vi "Implementation of Fast imaq image encode and decode.vi"() -> ()   [LabVIEW 2020]
uses:
  <vilib>/vision/Image Controls.llb/IMAQ Image.ctl
  <vilib>/NI/Tools/String/Tools_String.lvlib
  <vilib>/Analysis/NI_AALBase.lvlib
panel:
  out "Percent":dbl
  out "length1":i32
  out "length2":i32
  in  "TIFF Options":T1={"Rows Per Strip"=0, "Photometric"=1, "Compression Type"=0} {"Compression Type" items=["None", "JPEG", "Run Length Encoded", "Zip"]; "Photometric" items=["WhiteIsZero", "BlackIsZero"]}
  out "variance 2":dbl format="%0.2f"
  out "standard deviation 2":dbl format="%0.2f"
  out "mean 2":dbl format="%0.2f"
  out "variance":dbl format="%0.2f"
  out "standard deviation":dbl format="%0.2f"
  out "mean":dbl format="%0.2f"
  out "Array 1":u32[](array[numeric])
  out "Array":u32[](array[numeric])
  in  "Image Quality 2":u32=750 caption="Image Quality" max=1000 step=10
  out "FileString 2":string
  out "Y Resolution":i32
  out "X Resolution":i32
  in  "file (use dialog)":path
  out "FileString":string
  in  "Image Quality":u32=750 max=1000 step=10
  in  "File Options":T2 {"Optional Max Value" format="%.2f"; "Optional Min Value" format="%.2f"; "File Data Type" items=["1 bit", "2 bits", "4 bits", "8 bits", "16 bits (unsigned)", "16 bits (signed)", "16 bits (RGB chunky)", "24 bits (RGB chunky)", "24 bits (RGB planar)", "32 bits (unsigned)", "32 bits (signed)", "32 bits (RGB chunky)", "32 bits (float)", "48 bits (Complex 2x24 int)", "64 bits (Complex 2x32 float)", "32 bits (HSL)"]; "Read Raw File" items=["Don't Read Raw File ", "Read Raw File"]}
  in  "File Path":path
  in  "Image":T3
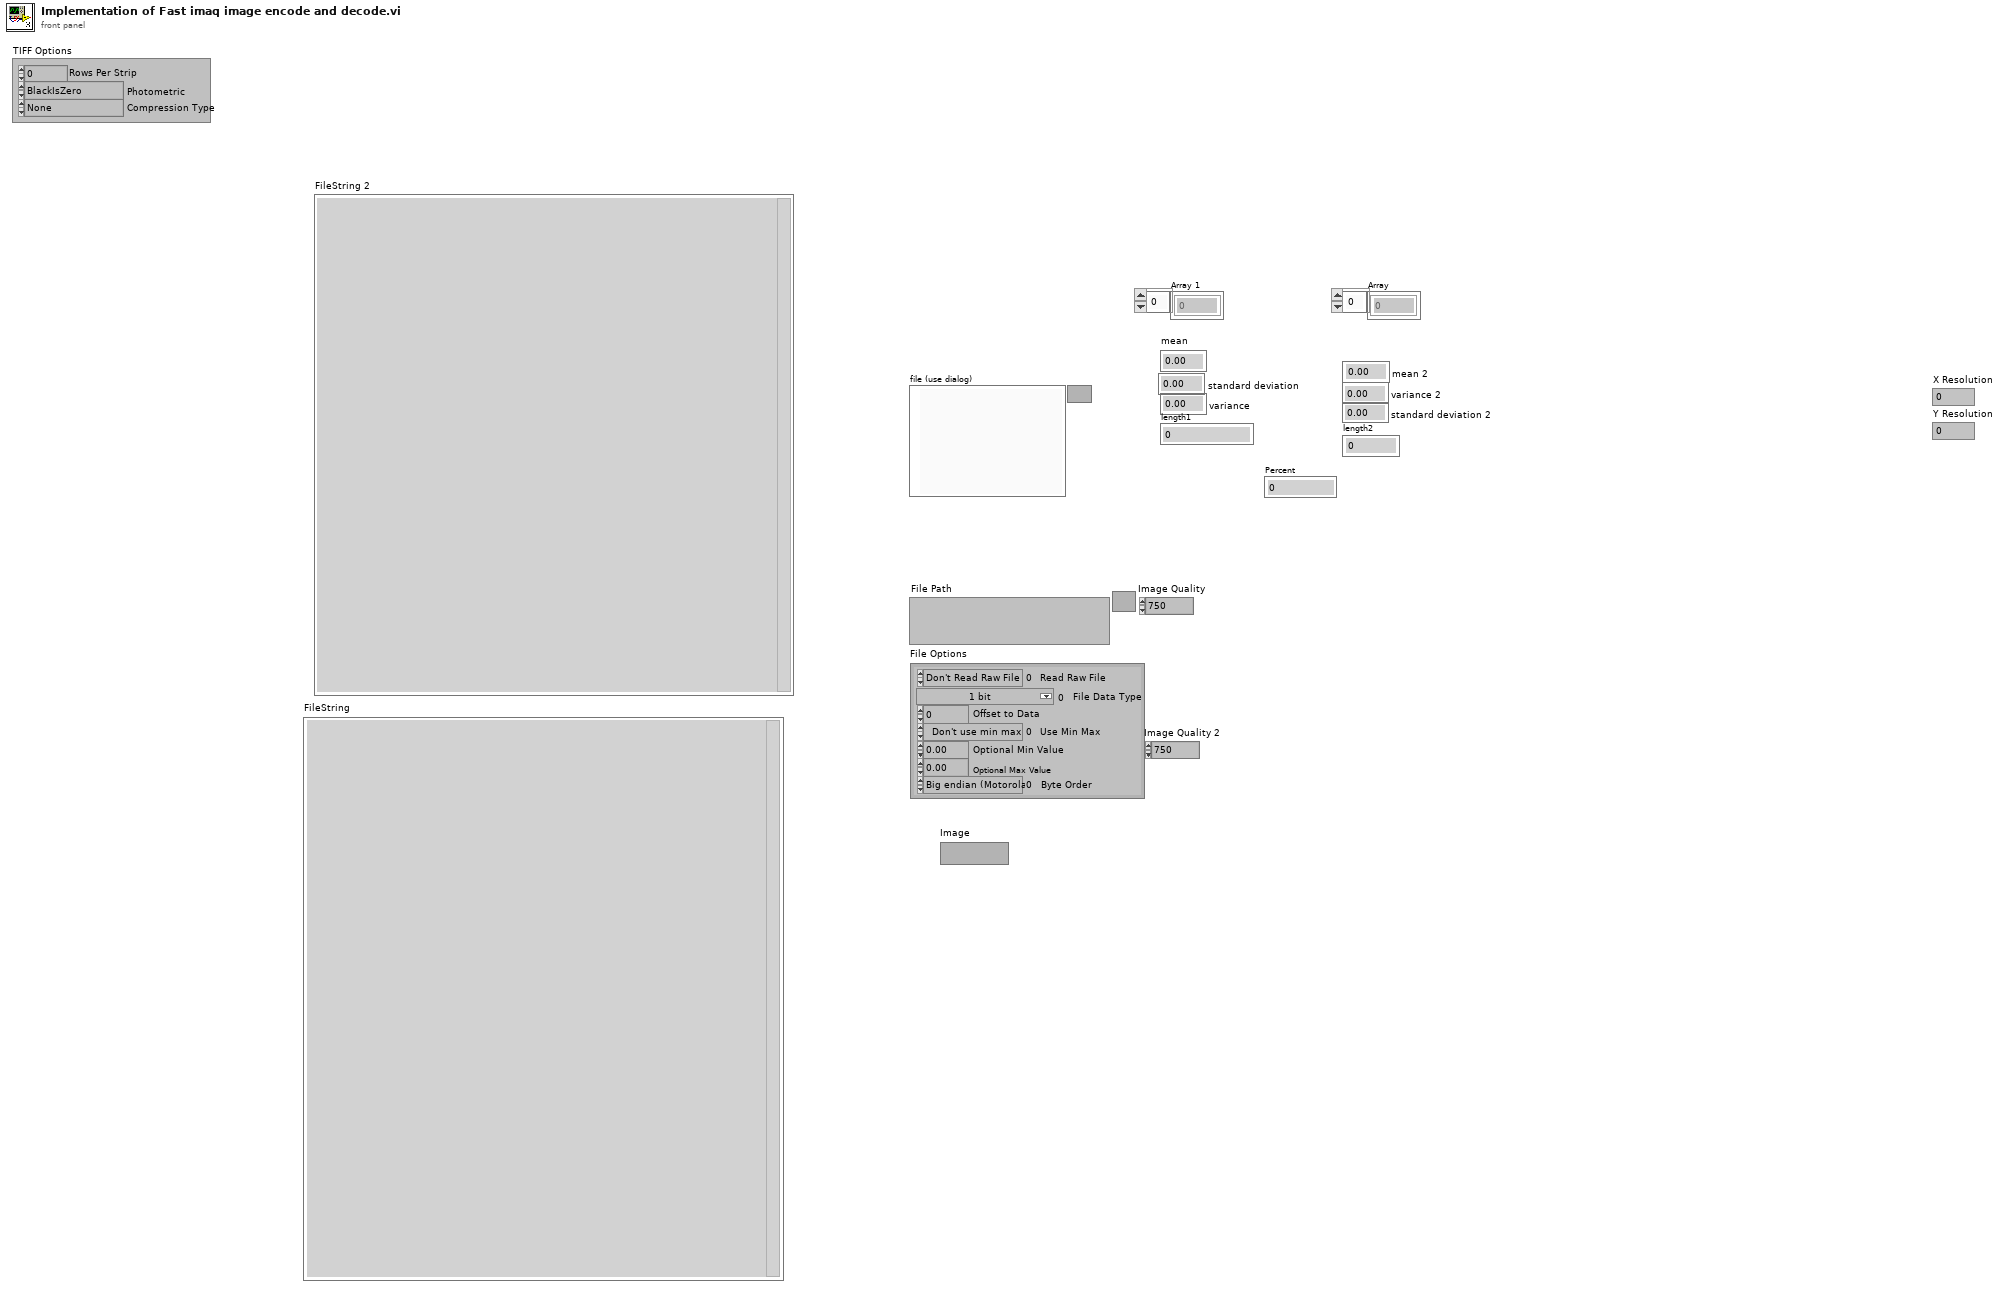
[diagram p1: front panel]
types:
  T1 = cluster{"Rows Per Strip":i32, "Photometric":i32, "Compression Type":i32}
  T2 = cluster{"Read Raw File":i32, "File Data Type":u32, "Offset to Data":i32, "Use Min Max":enum32{"Don't use min max", "Use file values", "Use optional values"}, "Optional Min Value":sgl, "Optional Max Value":sgl, "Byte Order":enum32{"Big endian (Motorola)", "Little endian (Intel)"}}
  T3 = typedef "IMAQ Image.ctl" = refnum<image>
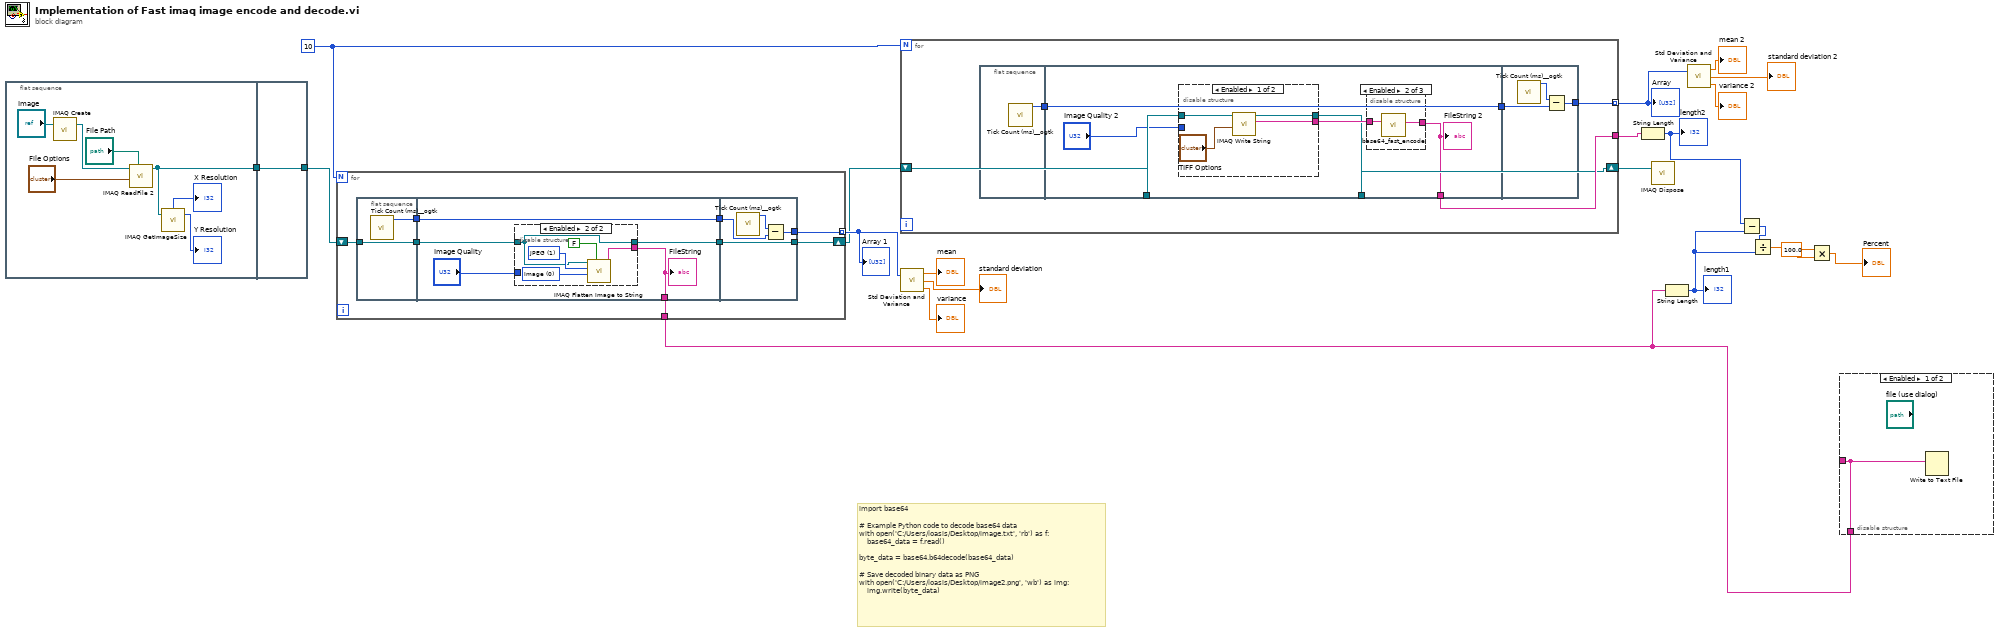
[diagram p0: block diagram]
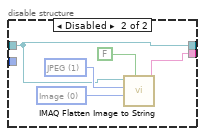
[diagram p3: hidden frame]
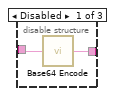
[diagram p4: hidden frame]
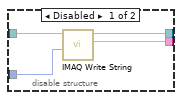
[diagram p6: hidden frame]
diagram:
  w18 = 10
  # "import base64\n\n# Example Python code to decode base64 data\nwith open('C:/Users/loasis/Desktop/image.txt', 'rb') as f:\n    base64_data = f.read()\n\nbyte_data = base64.b64decode(base64_data)\n\n# Save decoded binary data as PNG\nwith open('C:/Users/loasis/Desktop/image2.png', 'wb') as img:\n    img.write(byte_data)"
  n1 = flat-sequence {
    tunnel: [w22] -> w20
    tunnel: [w29] -> w21
    tunnel: w20 -> [w29]
    frame #0 {
      n2 = call "IMAQ Create"("Image Name"="Image") -> ("New Image"=w25:T3)  [unwired: 4 in, 1 out]
      n3 = call "IMAQ ReadFile 2"("File Path"="File Path", "File Options"="File Options", "Image"=w25) -> ("Image Out"=w22:T3)  [unwired: 4 in, 4 out]
      n4 = call "IMAQ GetImageSize"("Image"=w22) -> ("Y Resolution"=→"Y Resolution":i32, "X Resolution"=→"X Resolution":i32)  [unwired: 3 in, 1 out]
    }
    frame #1 {
    }
  }
  n5 = for {
    N: w18 -> [_]
    tunnel: [w31] -> w17 mode=indexing
    shift-right: [w36] -> w9
    shift-left: w21 -> [w37]
    tunnel: [w30] -> w7
    n6 = flat-sequence {
      tunnel: w37 -> [w39]
      tunnel: [w39] -> w35
      tunnel: [w38] -> w32
      tunnel: w35 -> [w43]
      tunnel: [w42] -> w34
      tunnel: [w41] -> w33
      tunnel: w32 -> [w41]
      tunnel: [w40] -> w30
      tunnel: [w57] -> w36
      tunnel: w34 -> [w57]
      tunnel: w33 -> [w56]
      tunnel: [w54] -> w31
      frame #0 {
        n7 = call <userlib>:"Tick Count (ms)__ogtk.vi"() -> ("millisecond timer value"=w38:u32)  [unwired: 10 in, 1 out]
      }
      frame #1 {
        n8 = disable-structure shown="Enabled" {
          disable-tunnel: "Image Quality" -> [w48 _]
          disable-tunnel: [w47 w50] -> w40
          disable-tunnel: w43 -> [w46 w49]
          disable-tunnel: [w45 w49] -> w42
          frame Disabled {
            n9 = call-poly "IMAQ Write String"("Image Quality"=w48, "Image"=w46) -> ("FileString"=w47:string, "Image Out (duplicate)"=w45:T3)  [unwired: 7 in, 1 out]
          }
          frame Enabled {
            w51 = 1 items=["None", "JPEG", "PACKED BINARY"] ("Compression (None)")
            w52 = 0 items=["Image", "Image and Vision Info", "Reference to Image"] ("Type of Flatten (Image and Vision Info)")
            n10 = call "IMAQ Flatten Image to String"("Flatten with Process-Unique Name (F)"=FALSE, "Type of Flatten (Image and Vision Info)"=w52, "Compression (None)"=w51, "Image"=w49) -> ("Data String"=w50:string)  [unwired: 6 in, 1 out]
          }
        }
        "FileString" <- w40
      }
      frame #2 {
        n11 = call <userlib>:"Tick Count (ms)__ogtk.vi"() -> ("millisecond timer value"=w55:u32)  [unwired: 10 in, 1 out]
        n12 = Subtract(x=w55, y=w56) -> (x-y=w54:u32)
      }
    }
  }
  "Array 1" <- w17
  n13 = for {
    N: w18 -> [_]
    tunnel: [w62] -> w8
    tunnel: [w58] -> w13 mode=indexing
    shift-right: [w61] -> w19
    shift-left: w9 -> [w63]
    n14 = flat-sequence {
      tunnel: [w64] -> w59
      tunnel: w63 -> [w70]
      tunnel: [w67] -> w62
      tunnel: [w66] -> w61
      tunnel: [w65] -> w60
      tunnel: w59 -> [w65]
      tunnel: w60 -> [w87]
      tunnel: [w85] -> w58
      frame #0 {
        n15 = call <userlib>:"Tick Count (ms)__ogtk.vi"() -> ("millisecond timer value"=w64:u32)  [unwired: 10 in, 1 out]
      }
      frame #1 {
        n16 = disable-structure shown="Enabled" {
          disable-tunnel: w70 -> [w74 w77]
          disable-tunnel: [w73 w76] -> w69
          disable-tunnel: "Image Quality 2" -> [_ _]
          disable-tunnel: [w72 w77] -> w66
          frame Enabled {
            n17 = call-poly "IMAQ Write String"("TIFF Options"="TIFF Options", "Image"=w74) -> ("FileString"=w73:string, "Image Out (duplicate)"=w72:T3)  [unwired: 7 in, 1 out]
          }
          frame Disabled {
            w78 = 1 items=["None", "JPEG", "PACKED BINARY"] ("Compression (None)")
            w79 = 0 items=["Image", "Image and Vision Info", "Reference to Image"] ("Type of Flatten (Image and Vision Info)")
            n18 = call "IMAQ Flatten Image to String"("Flatten with Process-Unique Name (F)"=FALSE, "Type of Flatten (Image and Vision Info)"=w79, "Compression (None)"=w78, "Image"=w77) -> ("Data String"=w76:string)  [unwired: 6 in, 1 out]
          }
        }
        n19 = disable-structure shown="Enabled" {
          disable-tunnel: w69 -> [w81 w83 w84]
          disable-tunnel: [w80 w82 w84] -> w67
          frame Disabled {
            n20 = call <vilib>:"Base64 Encode.vi"("normal string"=w81) -> ("base64 string"=w80:string)  [unwired: 1 in]
          }
          frame Enabled {
            n21 = call "base64_fast_encode.vi"("string in (not encoded)"=w83) -> ("string out (base64-encoded)"=w82:string)  [unwired: 9 in, 1 out]
          }
          frame Disabled {
          }
        }
        "FileString 2" <- w67
      }
      frame #2 {
        n22 = call <userlib>:"Tick Count (ms)__ogtk.vi"() -> ("millisecond timer value"=w86:u32)  [unwired: 10 in, 1 out]
        n23 = Subtract(x=w86, y=w87) -> (x-y=w85:u32)
      }
    }
  }
  "Array" <- w13
  n24 = call <vilib>:"Std Deviation and Variance.vi"("X"=w17) -> ("mean"=→"mean":dbl, "standard deviation"=→"standard deviation":dbl, "variance"=→"variance":dbl)  [unwired: 1 in]
  n25 = String Length(string=w8) -> (length=w6:i32)
  "length2" <- w6
  n26 = call "IMAQ Dispose"("Image"=w19) -> ()  [unwired: 5 in, 1 out]
  n27 = String Length(string=w7) -> (length=w4:i32)
  "length1" <- w4
  n28 = call <vilib>:"Std Deviation and Variance.vi"("X"=w13) -> ("mean"=→"mean 2":dbl, "standard deviation"=→"standard deviation 2":dbl, "variance"=→"variance 2":dbl)  [unwired: 1 in]
  n29 = Subtract(x=w6, y=w4) -> (x-y=w5:i32)
  n30 = Divide(x=w5, y=w4) -> (x/y=w3:dbl)
  n31 = Multiply(x=100.0, y=w3) -> (x*y=→"Percent":dbl)
  n32 = disable-structure shown="Enabled" {
    disable-tunnel: [w88 _] -> _
    disable-tunnel: w7 -> [w88 _]
    frame Enabled {
      n33 = Write to Text File(text=w88) -> ()  [unwired: 3 in, 3 out]
    }
    frame Disabled {
    }
  }
